vi "AlliGator Compute Optimal IRF v2.vi"(0 "Selected Plot Info":T8={"Multiplot XY Graph"=refnum, "Mouse Coordinates"={"Horizontal"=0, "Vertical"=0}, "Plot Index"=-1}, 5 "IRF*PSED Fixed Parameters":T3={"order"=0, "T"=0.0, "Time Constant Array"=[], "{S_k, C_k, phi_k, e_k} arrays"={"S_k Array"=[], "C_k Array"=[], "phi_k Array"=[], "e_k Array"=[]}, "IRF Extraction Options"={"Time Constant for IRF Extraction"=1e-18, "IRF Order"=0, "Fourier Series Smoothing"=enum."None", "Noise Threshold"=0.0, "Smoothing Width"=0.0, "Fourier Series Truncation"=enum."Automatic", "Truncation Order"=0, "Save Power Spectrum"=FALSE, "Smoothing"=FALSE, "Smoothing Parameter"=0.0, "Smoothing Order"=1, "Method"=enum."Direct"}} {"IRF Extraction Options"."Smoothing Order" min=1 max=10; "IRF Extraction Options"."Time Constant for IRF Extraction" format="%#_5g"}, 9 "IRF Optimization Control":T1={"Search Range"=1e-18, "Search Step"=1e-18, "Tail Threshold (%)"=1e-09, "Regularized IRF"=FALSE, "Export Plot"=FALSE, "Export Data"=FALSE, "Smooth Metrics"=FALSE, "S-G Side Points"=1, "S-G Polynomial Order"=3, "Metrics"=enum."Average"} {"S-G Polynomial Order" min=3 max=10; "S-G Side Points" min=1; "Tail Threshold (%)" min=0.0 max=100.0; "Search Range" min=0.0 max=1e-09}, 11 "Error In":errorcluster) -> (2 "Optimization Graph":cluster{"Ramp Pattern":dbl[], dbl[]}[](graph), 3 "Residuals Plot":cluster{"X Array":dbl[], "Y Array":dbl[]}, 4 "Fitted Plot":cluster{"X Array":dbl[], "Y Array":dbl[]}, 6 "Plot Name":string, 8 "Fit Parameter Values":dbl[](array[numeric]), 10 "Optimal Tau":dbl, 13 "Additional Data":variant, 14 "Fit Results String":string, 15 "Error Out":errorcluster)   [LabVIEW 2021, in "AlliGator Decay Analysis.lvlib" / "AlliGator IRF.lvlib"]
doc: "Extract IRF from provided decay using deconvolution and finding the minimal metrics."
uses:
  AlliGator IRF.lvlib
  Graphs/XY Graph/XY Graph Selected Plot Info.ctl
  Graphs/XY Graph/XY Graph Refnum.ctl
  <vilib>/Utility/miscctls.llb/LVPoint32TypeDef.ctl
  Fits/IRF(X)PSED/IRF(X)PSED Fixed Parameters v3.ctl
  Fits/IRF(X)PSED/IRF(X)PSED Extraction Options.ctl
  Fits/IRF(X)PSED/Fourier Series Smoothing Option.ctl
  Fits/IRF(X)PSED/Fourier Series Truncation.ctl
  Fits/IRF(X)PSED/IRF Extraction Method.ctl
  AlliGator IRF Optimization Controls.ctl
  AlliGator IRF Deconvolution Metrics.ctl
  AlliGator Settings List.ctl
  Fits/IRF(X)PSED/Decay Fit Options v2.ctl
  Fits/Decay Convolution/Decay Model.ctl
  Fits/Residual Type.ctl
  Fits/IRF(X)PSED/Fit Weights Type.ctl
  Fits/Non-linear Fitting Method v2.ctl
  Fits/Fit Calculation Method.ctl
  Fits/Non-linear Fitting Algorithm.ctl
  Fits/Fit Settings.ctl
  Fits/Nonlinear Fit Method.ctl
  Fits/Ramp Type.ctl
  Fits/Fit Plot Request Information.ctl
  <vilib>/Utility/miscctls.llb/LVPointDoubleTypeDef.ctl
  Fits/Fit Models.ctl
  <vilib>/Analysis/6fits.llb/Curve Fitting Criteria.ctl
  Fits/D-Only Fixed Parameters.ctl
  Fits/IRF(X)PSED/IRF(X)PSED Fit Parameters.ctl
  <vilib>/Analysis/1siggen.llb/Ramp Pattern by Delta.vi
  <vilib>/Analysis/NI_AALBase.lvlib
  AlliGator Settings.lvlib
  Time/Time.lvlib
  Fits/Fits.lvlib
  <vilib>/Analysis/NI_AALPro.lvlib
  Error/Error.lvlib
  Utilities/Utilities.lvlib
  Graphs/XY Graph/XY Graph Add-Ons.lvlib
panel:
  in  "Minimum Type":enum16{"Integral", "Chi 2", "Product"}(ring)=enum."Chi 2"
  out "Current Tau (ns)":dbl format="%#_4g"
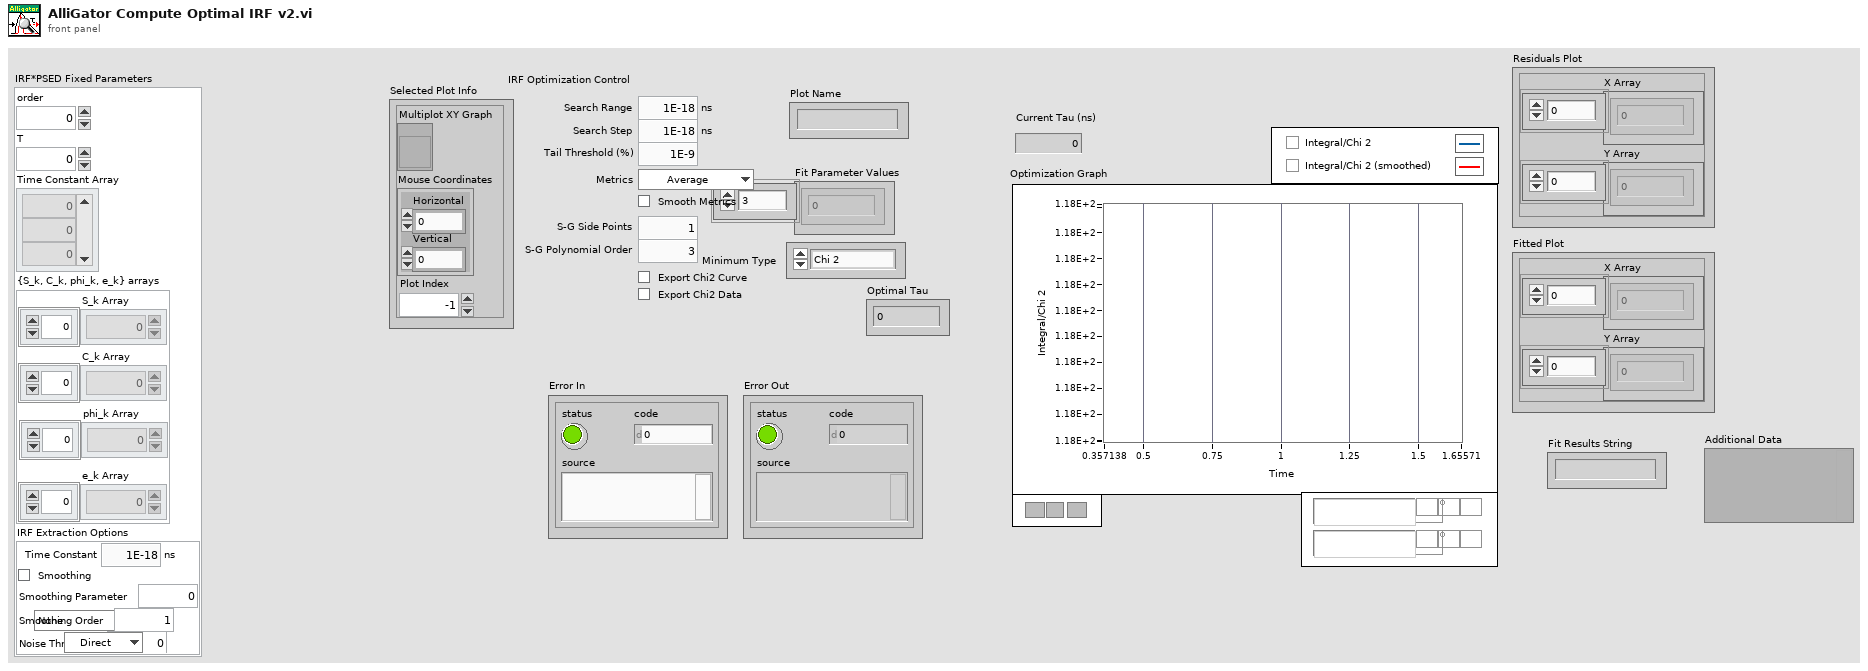
[diagram p1: front panel]
types:
  T1 = typedef "AlliGator Decay Analysis.lvlib/AlliGator IRF.lvlib/AlliGator IRF Optimization Controls.ctl" = cluster{"Search Range":dbl[unit], "Search Step":dbl[unit], "Tail Threshold (%)":dbl, "Regularized IRF":bool, "Export Plot":bool, "Export Data":bool, "Smooth Metrics":bool, "S-G Side Points":i32, "S-G Polynomial Order":i32, "Metrics":T2}
  T2 = typedef "AlliGator Decay Analysis.lvlib/AlliGator IRF.lvlib/AlliGator IRF Deconvolution Metrics.ctl" = enum16{"Average", "SDV", "Max", "Average * SDV", "Slope"}
  T3 = typedef "Fits.lvlib/IRF(X)PSED Fixed Parameters v3.ctl" = cluster{"order":i32, "T":dbl, "Time Constant Array":dbl[], "{S_k, C_k, phi_k, e_k} arrays":cluster{"S_k Array":dbl[], "C_k Array":dbl[], "phi_k Array":dbl[], "e_k Array":dbl[]}, "IRF Extraction Options":T4}
  T4 = typedef "Fits.lvlib/IRF(X)PSED Extraction Options.ctl" = cluster{"Time Constant for IRF Extraction":dbl[unit], "IRF Order":i32, "Fourier Series Smoothing":T5, "Noise Threshold":dbl, "Smoothing Width":dbl, "Fourier Series Truncation":T6, "Truncation Order":i32, "Save Power Spectrum":bool, "Smoothing":bool, "Smoothing Parameter":dbl, "Smoothing Order":u32, "Method":T7}
  T5 = typedef "Fits.lvlib/Fourier Series Smoothing Option.ctl" = enum16{"None", "Lanczos Factors", "Fejer Summation"}
  T6 = typedef "Fits.lvlib/Fourier Series Truncation.ctl" = enum16{"Automatic", "Fixed"}
  T7 = typedef "Fits.lvlib/IRF Extraction Method.ctl" = enum16{"Direct", "Topless", "Toeplitz"}
  T8 = typedef "XY Graph Add-Ons.lvlib/XY Graph Selected Plot Info.ctl" = cluster{"Multiplot XY Graph":T9, "Mouse Coordinates":T10, "Plot Index":i32}
  T9 = typedef "XY Graph Add-Ons.lvlib/XY Graph Refnum.ctl" = refnum<vi>
  T10 = typedef "LVPoint32TypeDef.ctl" = cluster{"Horizontal":i32, "Vertical":i32}
  T11 = typedef "Fits.lvlib/Fit Settings.ctl" = cluster{"Use Original Plot # Points":bool, "# Fit Plot Points":u32, "Fitting Method":T12, "Weighted Fit":bool, "Show All Fit Components":bool, "Axis Type":T13, "Show Fit Residuals":bool, "Residual Type":T14, "Fitting Algorithm":T15}
  T12 = typedef "Fits.lvlib/Nonlinear Fit Method.ctl" = enum16{"Least Square", "Least Absolute Residual", "Bisquare", "MLE"}
  T13 = typedef "Fits.lvlib/Ramp Type.ctl" = u16
  T14 = typedef "Fits.lvlib/Residual Type.ctl" = enum16{"Standard", "Normalized", "Reduced"}
  T15 = typedef "Fits.lvlib/Non-linear Fitting Algorithm.ctl" = enum16{"Levenberg-Marquardt", "Trust-Region Dogleg"}
  T16 = typedef "Fits.lvlib/Decay Fit Options v2.ctl" = cluster{"Show Fit Residuals":bool, "Fit Model":T17, "Residual Type":T14, "Max Decay Percentile":dbl, "Min Decay Percentile":dbl, "Show Full Decay":bool, "Weights":T18, "Fitting Method":T19, "Compute Parameter Uncertainties":bool, "Periodic Boundaries":bool, "Model Calculation":T20, "Period":dbl[unit], "Termination Criteria":cluster{"Max Iterations":i32, "Max Function Calls":i32, "Max Time":dbl[unit], "Function Tolerance":dbl, "Parameter Tolerance":dbl, "Gradient Tolerance":dbl, "Min Lambda":dbl, "Max Lambda":dbl, "Initial Tick Count":u32}, "Offset Resolution":dbl[unit], "Use Local IRF":bool, "Fitting Algorithm":T15}
  T17 = typedef "Fits.lvlib/Decay Model.ctl" = enum16{"1-Exponential", "2-Exponentials"}
  T18 = typedef "Fits.lvlib/Fit Weights Type.ctl" = enum16{"Unweighted", "1/Variance", "Best of All"}
  T19 = typedef "Fits.lvlib/Non-linear Fitting Method v2.ctl" = enum16{"Least Square", "Least Absolute Residual", "Bisquare", "MLE", "-", "Best of All"}
  T20 = typedef "Fits.lvlib/Fit Calculation Method.ctl" = enum16{"Simulation", "Convolution", "Integration"}
  T21 = typedef "AlliGator Settings.lvlib/AlliGator Settings List.ctl" = enum16{"GUI:Visible Settings Tab", "GUI:Last Run Version", "Source Image:Use Image Histogram for Contrast", "Source Image:Low Count Pixels Rejection Options", "Source Image:High Count Pixels Rejection Options", "Source Image:Use Image Brightness", "Source Image:Blend Overlay with Image Background", "Source Image:Use Fixed ROI Diameter", "Source Image:ROI Diameter", "Source Image:ROI Center Color", "Source Image:Peak Threshold", "Source Image:Intensity Threshold", "Source Image:Image Binning Options", "Source Image:Image Smoothing Options", "Source Image:Image Histogram Active", "Source Image:Invert Binary Mask", "Source Image:Hot Pixel Removal", "Source Image:Overlay Analyzed ROI Center", "Source Image:Auto-Adjust Contrast", "Source Image:Histogram Lower Percentile", "Source Image:Histogram Upper Percentile", "Source Image:Save Source Image", "Source Image:Scale Bar Options", "Source Image:Image Resolution (Pixel Size)", "Source Image:Flatfield Correction", "Source Image:Show Dead Left Columns Correction", "Source Image:Dead Left Columns Correction", "Source Image:Image Pre-Processing Operations Order", "Source Image:Overlay ROI Median", "Source Image:Median Overlay Color", "Data Information:Gate Width", "Data Information:Nanotime Gate Separation", "Data Information:Macrotime Gate Separation", "Data Information:Gate Step", "Data Information:# Gates", "Data Information:Gate Image Exposure", "Data Information:Gate Image Integration", "Data Information:Gates to Skip", "Data Information:Gates to Keep", "Data Information:Define Gates to", "Data Information:Channel Name", "Data Information:Available Channel Names", "Data Information:Channel Arithmetic", "Data Information:Background File Subtraction", "Data Information:Background File", "Data Information:Background Scaling Factor", "Data Information:Background Pile-up Correction", "Data Information:Background Pixel Well Capacity", "Data Information:Laser Period", "Data Information:SYNC Period", "Data Information:Pile-up Correction", "Data Information:Pixel Well Capacity", "Data Information:Dataset Scaling Factor", "Fluorescence Decay_Decay Pre-Processing:Reverse Gates", "Fluorescence Decay_Decay Pre-Processing:Verbose Decay Pre-Processing", "Fluorescence Decay_Decay Pre-Processing:Use Decay Pre-Processing", "Fluorescence Decay_Decay Pre-Processing:Background Subtraction", "Fluorescence Decay_Decay Pre-Processing:Background Definition Range", "Fluorescence Decay_Decay Pre-Processing:Baseline Subtraction Method", "Fluorescence Decay_Decay Pre-Processing:Decay Pre-Processing Operations Order", "Fluorescence Decay_Decay Pre-Processing:Smoothing Parameter", "Fluorescence Decay_Decay Pre-Processing:Shift Decay", "Fluorescence Decay_Decay Pre-Processing:Decay Shift Parameters", "Fluorescence Decay_Decay Pre-Processing:Fold Decay", "Fluorescence Decay_Decay Pre-Processing:# Folds", "Fluorescence Decay_Decay Pre-Processing:1-Normalize Decay", "Fluorescence Decay_Decay Pre-Processing:[0-1]-Normalize Decay", "Fluorescence Decay_Decay Pre-Processing:Smoothen Decay", "Fluorescence Decay_Decay Pre-Processing:Extrapolate Decay", "Fluorescence Decay_Decay Pre-Processing:Use Periodicity", "Fluorescence Decay_Decay Pre-Processing:Use Cursors", "Fluorescence Decay_Decay Pre-Processing:Tail Fraction", "Fluorescence Decay_Decay Pre-Processing:Head Fraction", "Fluorescence Decay_Decay Pre-Processing:Additional Points", "Fluorescence Decay_Decay Pre-Processing:Straighten Decay", "Fluorescence Decay_Decay Pre-Processing:Constant Background", "Fluorescence Decay_Decay Pre-Processing:Pixel-Normalize Decay", "Fluorescence Decay_Advanced Analysis:Extract IRF instead of Decay", "Fluorescence Decay_Advanced Analysis:IRF Extraction Options", "Fluorescence Decay_Advanced Analysis:IRF Optimization Options", "Fluorescence Decay_Advanced Analysis:Square Pulse Options", "Fluorescence Decay_Advanced Analysis:IRF Order", "Fluorescence Decay_Advanced Analysis:IRF Time Constants", "Fluorescence Decay_Advanced Analysis:Wavelet Analysis Options", "Fluorescence Decay_Advanced Analysis:Average Lifetime Options", "Fluorescence Decay_Fit Options:Fit Options", "Fluorescence Decay_Fit Options:Use Legacy Fitting Approach", "Fluorescence Decay_Fit Options:Use Data Information Laser Period", "Fluorescence Decay_Fit Parameters:Displayed Fit Parameters", "Fluorescence Decay_Fit Parameters:Fit Parameter Constraints", "Fluorescence Decay_Fit Parameters:Export Tabulated Results", "Fluorescence Decay_Fit Parameters:MLE Baseline Offset Type", "Fluorescence Decay_Fit Parameters:MLE Baseline Offset", "Fluorescence Decay_Fit Parameters:Guess Parameter Names", "Fluorescence Decay_Fit Parameters:Guess Parameter Values", "Fluorescence Decay_Fit Parameters:Guess Parameters Options", "Fluorescence Decay_Styles:Show Last Decay Only", "Fluorescence Decay_Styles:Decay Graph Color Array", "Fluorescence Decay:Decay Graph Active", "Fluorescence Decay Statistics:Min Peak Value", "Fluorescence Decay Statistics:Reject Low Decay Peak Pixels", "Fluorescence Decay Statistics:Reject High Decay Peak Pixels", "Fluorescence Decay Statistics:Max Peak Value", "Time Traces:Use File Timestamp", "Time Traces:Time Step", "Time Traces:Use Intensity Correction File", "Time Traces:Intensity Correction File", "Phasor Plot:Phasor Plot Smoothing Options", "Phasor Plot:Phasor Plot Size", "Phasor Plot:Phasor Plot Graphics Options", "Phasor Plot:Cumulative Phasor Plot", "Phasor Plot:Use Phasor Brightness", "Phasor Plot:Blend Overlay with Phasor Background", "Phasor Plot:Save Phasor Plot", "Phasor Plot:Show References", "Phasor Plot:Phasor Ratio Decay Range", "Phasor Plot:Exponential Fading", "Phasor Plot:Phasor Ratio Reference Colors", "Phasor Plot:Reference Radius", "Phasor Plot:Show Color Map Vertices", "Phasor Plot:Phasor Plot Active", "Phasor Plot:Phasor Ratio Color Map Type", "Phasor Plot:Phasor Ratio Color Map", "Phasor Plot:Phasor Ratio Display Range", "Phasor Plot:Selected Image ROI(s)", "Phasor Plot:All Image ROIs", "Phasor Plot:Selected Phasor Plot ROI(s)", "Phasor Plot:All Phasor Plot ROIs", "Phasor Plot:Phasor Ratio Color-Coded Quantity", "Phasor Plot:Store Phasor Harmonics", "Phasor Plot:Draw Reference Segment", "Phasor Plot:User-Defined Quantity", "Phasor Graph:Phasor Frequency", "Phasor Graph:Phasor Ratio Type", "Phasor Graph:Pixel-level Phasor Computation", "Phasor Graph:Save Phasor Graph", "Phasor Graph:Phasor Graph Active", "Phasor Graph:Phasor SDV Options", "Phasor Calibration:Use Backup Calibration if needed", "Phasor Graph:Define Shortest Lifetime as", "Phasor Calibration:Backup Calibration Type", "Phasor Calibration:Calibration Type", "Phasor Calibration:Calibration Lifetime", "Phasor Calibration:Calibration Map Algorithm", "Single-Exponential Phasor Locus (SEPL):Gate Parameters", "Single-Exponential Phasor Locus (SEPL):User-defined Gate", "Single-Exponential Phasor Locus (SEPL):User-defined IRF", "Single-Exponential Phasor Locus (SEPL):Phasor Parameters", "Single-Exponential Phasor Locus (SEPL):Decay & IRF Parameters", "Single-Exponential Phasor Locus (SEPL):Display Parameters", "Lifetime Analysis:Decay Analysis Parameters", "Lifetime Analysis:Lifetime Map Active", "Plugins:Python Settings", "Miscellaneous:Verbose Mode", "Miscellaneous:Beep after Script", "Miscellaneous:Saved Image File Format", "Miscellaneous:Exported Gate Image Settings", "Miscellaneous:Include Loading in Timing", "Miscellaneous:Verbose Settings Mode", "Miscellaneous:Histogram Options", "Miscellaneous:Beep on Error", "Miscellaneous:# Logical Processors Used", "Miscellaneous:ROI Description Max Characters", "Miscellaneous:Verbose Error Mode", "Miscellaneous:Transparent Mask Color"}
  T22 = typedef "Fits.lvlib/Fit Plot Request Information.ctl" = cluster{"XY Graph Ref":refnum<vi>, "Mouse Coordinates":T23, "Fit Model":T24, "Plot Index":i32}
  T23 = typedef "LVPointDoubleTypeDef.ctl" = cluster{"X":dbl, "Y":dbl}
  T24 = typedef "Fits.lvlib/Fit Models.ctl" = enum16{"Select a Fit Model...", "           Single Peak", "Gaussian", "Asymmetric Gaussian", "Lorentzian", "Asymmetric Lorentzian", "Gaussian/Lorentzian", "Lorentzian/Gaussian", "           Double Peak", "Two Gaussians", "Two Asymmetric Gaussians", "Two H-Connected Gaussians", "Two T-Connected Gaussians", "Two H-Connected Asymmetric Gaussians", "Two T-Connected Asymmetric Gaussians", "           Triple Peak", "Three Gaussians", "Three Asymmetric Gaussians", "              Decays", "1-Exponential", "IRF*PSED", "2-Exponentials", "               ACF", "2D Gaussian ACF", "2D Gaussian + Blinking ACF", "2D Gaussian + Flow ACF", "3D Gaussian ACF", "3D Gaussian + Blinking ACF", "             Multiplot", "2D Gaussian ACF & 2D Gaussian + Flow ACF"}
  T25 = typedef "Fits.lvlib/IRF(X)PSED Fit Parameters.ctl" = cluster{"Offset":dbl, "Amplitudes":dbl[], "Time Constants":dbl[], "Baseline":dbl, "Lifetime":dbl, "IRF order":dbl, "Period":dbl, "SDV":dbl, "FWHM":dbl, "Integral":dbl, "MSE":dbl, "R^2":dbl}
  T26 = typedef "Fits.lvlib/D-Only Fixed Parameters.ctl" = cluster{"Fix D-only Peak Location":bool, "Peak Location":dbl, "Fix D-only Peak FWHM":bool, "Peak FWHM":dbl}
  T27 = typedef "NI_AALPro.lvlib/Curve Fitting Criteria.ctl" = u16
  T28 = cluster{"Ramp Pattern":dbl[], "Best Polynomial Fit":dbl[]}
  T29 = cluster{"Ramp Pattern":dbl[], "Best Polynomial Fit":dbl[]}[]
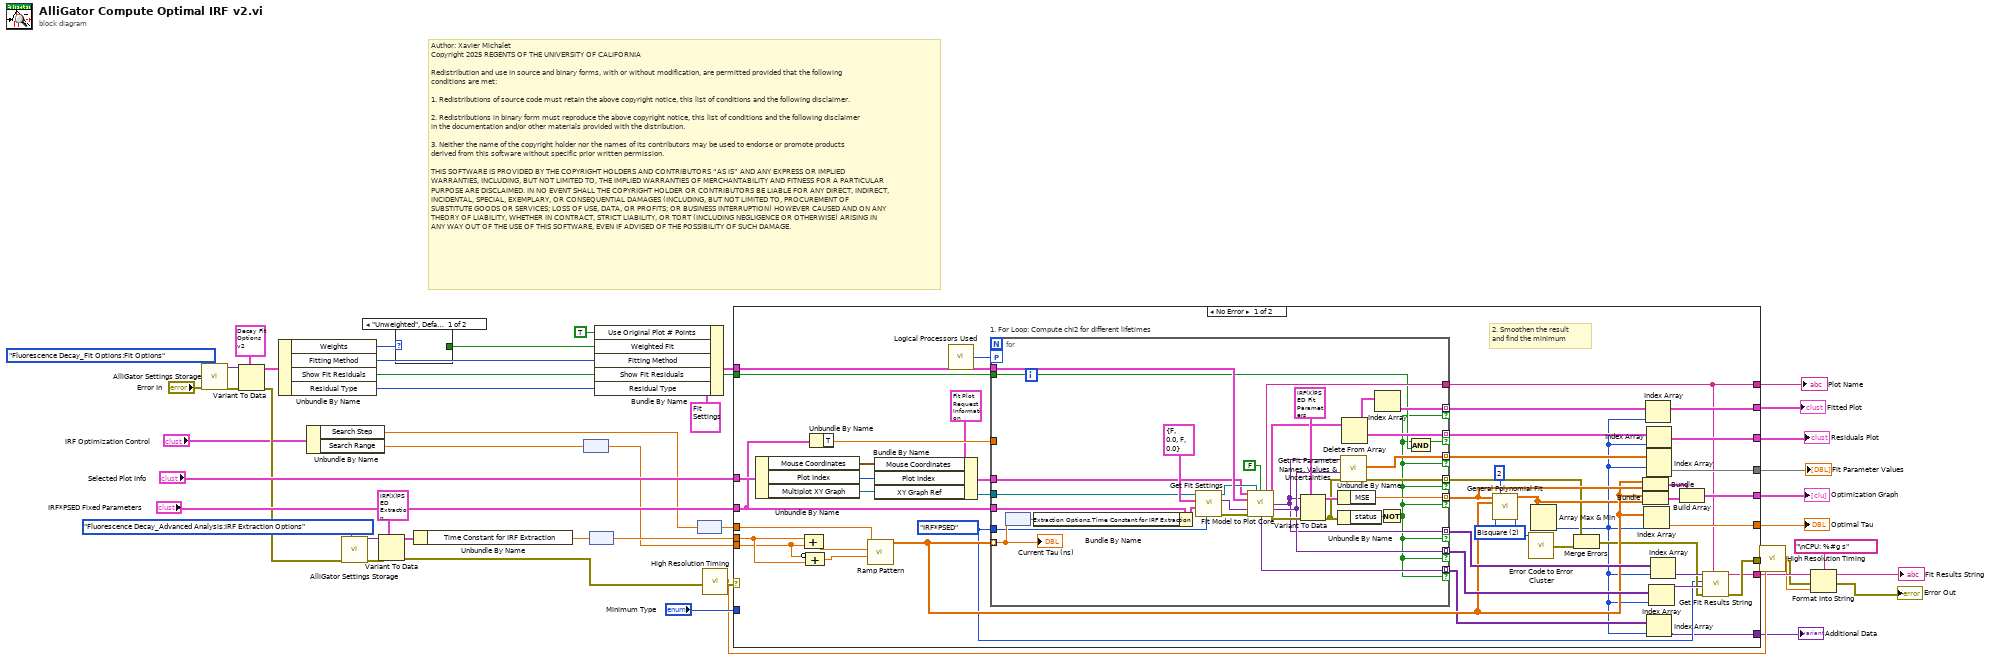
[diagram p0: block diagram]
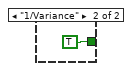
[diagram p2: hidden frame]
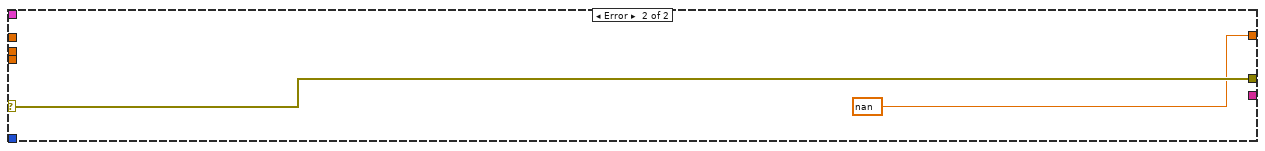
[diagram p3: hidden frame]
diagram:
  # "Author: Xavier Michalet\nCopyright 2025 REGENTS OF THE UNIVERSITY OF CALIFORNIA\n\nRedistribution and use in source and binary forms, with or without modification, are permitted provided that the following conditions are met:\n\n1. Redistributions of source code must retain the above copyright notice, this list of conditions and the following disclaimer.\n\n2. Redistributions in binary form must reproduce the above copyright notice, this list of conditions and the following disclaimer in the documentation and/or other materials provided with the distribution.\n\n3. Neither the name of the copyright holder nor the names of its contributors may be used to endorse or promote products derived from this software without specific prior written permission.\n\nTHIS SOFTWARE IS PROVIDED BY THE COPYRIGHT HOLDERS AND CONTRIBUTORS “AS IS” AND ANY EXPRESS OR IMPLIED WARRANTIES, INCLUDING, BUT NOT LIMITED TO, THE IMPLIED WARRANTIES OF MERCHANTABILITY AND FITNESS FOR A PARTICULAR PURPOSE ARE DISCLAIMED. IN NO EVENT SHALL THE COPYRIGHT HOLDER OR CONTRIBUTORS BE LIABLE FOR ANY DIRECT, INDIRECT, INCIDENTAL, SPECIAL, EXEMPLARY, OR CONSEQUENTIAL DAMAGES (INCLUDING, BUT NOT LIMITED TO, PROCUREMENT OF SUBSTITUTE GOODS OR SERVICES; LOSS OF USE, DATA, OR PROFITS; OR BUSINESS INTERRUPTION) HOWEVER CAUSED AND ON ANY THEORY OF LIABILITY, WHETHER IN CONTRACT, STRICT LIABILITY, OR TORT (INCLUDING NEGLIGENCE OR OTHERWISE) ARISING IN ANY WAY OUT OF THE USE OF THIS SOFTWARE, EVEN IF ADVISED OF THE POSSIBILITY OF SUCH DAMAGE."
  n1 = call "AlliGator Settings Storage.vi"("AlliGator Settings List"=AlliGator_Settings_List."Fluorescence Decay_Fit Options:Fit Options", "Error In"="Error In") -> ("Error Out"=w35:errorcluster, "Variant Data out"=w34:variant)  [unwired: 8 in]
  n2 = Variant To Data(error in=w35, type=T16 {"Show Fit Residuals"=TRUE, "Fit Model"=enum."1-Exponential", "Residual Type"=enum."Standard", "Max Decay Percentile"=0.0, "Min Decay Percentile"=0.0, "Show Full Decay"=TRUE, "Weights"=enum."Unweighted", "Fitting Method"=enum."Least Square", "Compute Parameter Uncertainties"=TRUE, "Periodic Boundaries"=TRUE, "Model Calculation"=enum."Simulation", "Period"=1.2500000000000001e-08, "Termination Criteria"={"Max Iterations"=1000, "Max Function Calls"=0, "Max Time"=1000.0, "Function Tolerance"=1e-06, "Parameter Tolerance"=1e-06, "Gradient Tolerance"=0.0, "Min Lambda"=1e-06, "Max Lambda"=1e-06, "Initial Tick Count"=0}, "Offset Resolution"=1.2500000000000001e-08, "Use Local IRF"=TRUE, "Fitting Algorithm"=enum."Levenberg-Marquardt"} ("Fit Options"), Variant=w34) -> (data=w32:T16, error out=w26:errorcluster)
  n3 = Unbundle By Name(w32) -> ("Weights"=w8:T18, "Fitting Method"=w30:T19, "Show Fit Residuals"=w16:bool, "Residual Type"=w29:T14)
  n4 = Unbundle By Name("IRF Optimization Control") -> ("Search Step"=w3:dbl[unit], "Search Range"=w2:dbl[unit])
  n5 = call "AlliGator Settings Storage.vi"("AlliGator Settings List"=AlliGator_Settings_List."Fluorescence Decay_Advanced Analysis:IRF Extraction Options", "Error In"=w26) -> ("Error Out"=w25:errorcluster, "Variant Data out"=w45:variant)  [unwired: 8 in]
  n6 = Variant To Data(error in=w25, type=T4 {"Time Constant for IRF Extraction"=1e-18, "IRF Order"=1, "Fourier Series Smoothing"=enum."None", "Noise Threshold"=0.0, "Smoothing Width"=0.0, "Fourier Series Truncation"=enum."Automatic", "Truncation Order"=0, "Save Power Spectrum"=FALSE, "Smoothing"=FALSE, "Smoothing Parameter"=0.0, "Smoothing Order"=1, "Method"=enum."Direct"} ("IRF Extraction Options"), Variant=w45) -> (data=w46:T4, error out=w24:errorcluster)
  n7 = case shown="\"Unweighted\", Default" w8 {
    tunnel: [_ TRUE ("Weighted Fit")] -> w7
    frame "Unweighted", Default {
    }
    frame "1/Variance" {
    }
  }
  n8 = Unbundle By Name(w46) -> ("Time Constant for IRF Extraction"=w5:dbl[unit])
  n9 = node(w2) -> (w1:dbl)
  n10 = node(w5) -> (w39:dbl)
  n11 = Bundle By Name(cluster=T11 {"Use Original Plot # Points"=TRUE, "# Fit Plot Points"=0, "Fitting Method"=enum."Least Square", "Weighted Fit"=FALSE, "Show All Fit Components"=FALSE, "Axis Type"=0, "Show Fit Residuals"=FALSE, "Residual Type"=enum."Standard", "Fitting Algorithm"=enum."Levenberg-Marquardt"} ("Fit Settings"), "Use Original Plot # Points"=TRUE, "Weighted Fit"=w7, "Fitting Method"=w30, "Show Fit Residuals"=w16, "Residual Type"=w29) -> (w28:T11)
  n12 = node(w3) -> (w40:dbl)
  n13 = call "High Resolution Timing.vi"("Error In"=w24) -> ("elapsed (relative) seconds"=w23:dbl, "Error Out"=w42:errorcluster)  [unwired: 16 in, 1 out]
  n14 = case shown="No Error" w42 {
    selector: w42 -> [_ w128]
    tunnel: [w65 w128] -> w47
    tunnel: w39 -> [w92 _]
    tunnel: [w84 nan] -> w43
    tunnel: "Minimum Type" -> [_ _]
    tunnel: w40 -> [w91 _]
    tunnel: w1 -> [w90 _]
    tunnel: "Selected Plot Info" -> [w87 _]
    tunnel: "IRF*PSED Fixed Parameters" -> [w86 _]
    tunnel: w28 -> [w88 _]
    tunnel: [w78 _] -> w22
    tunnel: [w64 _] -> w21
    tunnel: [w76 _] -> w20
    tunnel: [w74 _] -> w19
    tunnel: [w72 _] -> w17
    tunnel: w16 -> [w71 _]
    tunnel: [w63 _] -> w15
    tunnel: [w51 _] -> w9
    frame No Error {
      w60 = T27 2 items=["Least Square", "Least Absolute Residual", "Bisquare"] ("method")
      w54 = Fit_Models."IRF*PSED" ("Fit Model")
      # "2. Smoothen the result\nand find the minimum"
      n15 = Unbundle By Name(w87) -> ("Mouse Coordinates"=w80:T10, "Plot Index"=w79:i32, "Multiplot XY Graph"=w81:T9)
      n16 = Compound Arithmetic op=ADD(w92, w90) -> (w94:dbl)
      n17 = Compound Arithmetic op=ADD(invert w90, w92) -> (w93:dbl)
      n18 = Unbundle By Name(w86) -> ("T"=w85:dbl)
      n19 = call-poly <vilib>:"Ramp Pattern.vi"("start"=w93, "end"=w94, "delta"=w91) -> ("Ramp Pattern"=w61:dbl[])  [unwired: 6 in, 2 out]
      n20 = Bundle By Name(cluster=T22 {"XY Graph Ref"=refnum, "Mouse Coordinates"={"X"=0.0, "Y"=0.0}, "Fit Model"=enum."IRF*PSED", "Plot Index"=-1} ("Fit Plot Information"), "Mouse Coordinates"=w80, "Plot Index"=w79, "XY Graph Ref"=w81) -> (w82:T22)
      n21 = call "Logical Processors Used.vi"() -> ("# Logical Processor Used"=w49:i32)  [unwired: 6 in]
      n22 = for "1. For Loop: Compute chi2 for different lifetimes" {
        tunnel: w61 -> [w125] mode=indexing
        workers-P: w49 -> [_]
        tunnel: w88 -> [w121]
        tunnel: w86 -> [w126]
        tunnel: w81 -> [w112]
        tunnel: [w114] -> w62 mode=indexing if=w96
        tunnel: w85 -> [_]
        tunnel: w82 -> [w111]
        tunnel: [w110] -> w64
        tunnel: [w109] -> w77 mode=indexing if=w96
        tunnel: [w108] -> w55 mode=indexing if=w96
        tunnel: [w106] -> w75 mode=indexing if=w102
        tunnel: [w103] -> w73 mode=indexing if=w96
        tunnel: w71 -> [w101]
        tunnel: [w98] -> w69 mode=indexing if=w96
        tunnel: [w100] -> w68 mode=indexing if=w96
        tunnel: w54 -> [w99]
        tunnel: [w97] -> w53 mode=indexing if=w96
        n23 = node(w125) -> (w95:dbl[unit])
        n24 = Bundle By Name(cluster=w126, "IRF Extraction Options.Time Constant for IRF Extraction"=w95) -> (w124:T3)
        n25 = call "Get Fit Settings.vi"("Fit Model"=w99, "Additional Parameters"=w124, "Fixed Parameters"=T26 {"Fix D-only Peak Location"=FALSE, "Peak Location"=0.0, "Fix D-only Peak FWHM"=FALSE, "Peak FWHM"=0.0}, "XY Graph Ref"=w112) -> ("Error Out"=w122:errorcluster, "Additional Fit Settings"=w120:variant, "LM Function & Gradient"=w119:refnum<vi>)  [unwired: 5 in]
        n26 = call "Fit Model to Plot Core.vi"("Fit Plot Information"=w111, "LM Function & Gradient"=w119, "Display Plots (T)"=FALSE, "Fit Settings"=w121, "Additional Data (in)"=w120, "error in (no error)"=w122) -> ("Plot Name"=w110:string, "Array of Plots (Fit, Components, Residuals)"=w105:cluster{"X Array":dbl[], "Y Array":dbl[]}[], "Fit Parameters Cluster"=w98:variant, "Fit Parameters Uncertainties Cluster"=w100:variant, "Additional Data (out)"=w97:variant, "error out"=w116:errorcluster)  [unwired: 2 in, 2 out]
        n27 = Variant To Data(error in=w116, type=T25 {"Offset"=0.0, "Amplitudes"=[], "Time Constants"=[], "Baseline"=0.0, "Lifetime"=0.0, "IRF order"=0.0, "Period"=0.0, "SDV"=0.0, "FWHM"=0.0, "Integral"=0.0, "MSE"=0.0, "R^2"=0.0} ("IRF*PSED Fit Parameters"), Variant=w98) -> (data=w117:T25, error out=w113:errorcluster)
        n28 = Unbundle By Name(w117) -> ("MSE"=w114:dbl)
        n29 = Unbundle By Name(w113) -> ("status"=w115:bool)
        n30 = call "Get Fit Parameter Names, Values & Uncertainties.vi"("error in (no error)"=w113, "Fit Parameter Uncertainties"=w100, "Fit Parameters"=w98) -> ("Error Out"=w108:errorcluster, "Fit Parameter Values"=w109:dbl[])  [unwired: 5 in, 2 out]
        n31 = Delete From Array(array=w105) -> (deleted portion=w106:cluster{"X Array":dbl[], "Y Array":dbl[]}, array with subset deleted=w104:cluster{"X Array":dbl[], "Y Array":dbl[]}[])  [unwired: 2 in]
        n32 = Index Array(array=w104) -> (element=w103:cluster{"X Array":dbl[], "Y Array":dbl[]})  [unwired: 1 in]
        n33 = Not(x=w115) -> (.not. x?=w96:bool)
        n34 = Compound Arithmetic op=AND(w96, w101) -> (w102:bool)
        "Current Tau (ns)" <- w125
      }
      n35 = call <vilib>:"General Polynomial Fit.vi"("Y"=w62, "polynomial order"=2, "X"=w61, "method"=w60) -> ("Best Polynomial Fit"=w58:dbl[], "error"=w57:i32)  [unwired: 8 in, 2 out]
      n36 = call "Error Code to Error Cluster.vi"("Error Code"=w57) -> ("Error Out"=w50:errorcluster)  [unwired: 14 in]
      n37 = Array Max & Min(array=w58) -> (min index (indices)=w52:i32)  [unwired: 3 out]
      n38 = Merge Errors(w55, w50) -> (w56:errorcluster)
      n39 = Bundle("Ramp Pattern"=w61, w62) -> (w70:cluster{"Ramp Pattern":dbl[], dbl[]})  [unwired: 1 in]
      n40 = Bundle("Ramp Pattern"=w61, "Best Polynomial Fit"=w58) -> (w89:T28)  [unwired: 1 in]
      n41 = Index Array(array=w61, index=w52) -> (element=w84:dbl)
      n42 = Index Array(array=w73, index=w52) -> (element=w72:cluster{"X Array":dbl[], "Y Array":dbl[]})
      n43 = Index Array(array=w75, index=w52) -> (element=w74:cluster{"X Array":dbl[], "Y Array":dbl[]})
      n44 = Index Array(array=w77, index (row)=w52) -> (element=w76:dbl[])  [unwired: 1 in]
      n45 = Index Array(array=w53, index=w52) -> (element=w51:variant)
      n46 = Index Array(array=w68, index=w52) -> (element=w66:variant)
      n47 = Index Array(array=w69, index=w52) -> (element=w67:variant)
      n48 = Build Array(w70, w89) -> (w78:T29)
      n49 = call "Get Fit Results String.vi"("Plot Name"=w64, "error in (no error)"=w56, "Fit Parameters Uncertainties Cluster"=w66, "Fit Model"=w54, "Fit Parameters Cluster"=w67) -> ("error out"=w65:errorcluster, "Fit Results String"=w63:string)  [unwired: 5 in]
    }
    frame Error {
    }
  }
  "Optimal Tau" <- w43
  "Optimization Graph" <- w22
  "Plot Name" <- w21
  "Fit Parameter Values" <- w20
  "Residuals Plot" <- w19
  "Fitted Plot" <- w17
  "Additional Data" <- w9
  n50 = call "High Resolution Timing.vi"("relative seconds (NaN)"=w23, "Error In"=w47) -> ("elapsed (relative) seconds"=w13:dbl, "Error Out"=w11:errorcluster)  [unwired: 15 in, 1 out]
  n51 = Format Into String(format string="\nCPU: %#g s", initial string=w15, error in=w11, w13) -> (resulting string=→"Fit Results String":string, error out=→"Error Out":errorcluster)
